vi "Supplementary Fig.13.vi"() -> ()   [LabVIEW 2018]
uses:
  <vilib>/Utility/miscctls.llb/LVBoundsTypeDef.ctl
panel:
  out "files":string[](array[string])=["3rd-no3_th0_20191112171700-ext.FIRE", "3rd-no3_th0_20191112171706-ext.FIRE", "3rd-no3_th0_20191112171712-ext.FIRE", "3rd-no3_th0_20191112171717-ext.FIRE", "3rd-no3_th0_20191112171723-ext.FIRE", "3rd-no3_th0_20191112171728-ext.FIRE", "3rd-no3_th0_20191112171733-ext.FIRE", "3rd-no3_th0_20191112171739-ext.FIRE", "3rd-no3_th0_20191112171744-ext.FIRE", "3rd-no3_th0_20191112171750-ext.FIRE", "3rd-no3_th0_20191112171756-ext.FIRE", "3rd-no3_th0_20191112171801-ext.FIRE", "3rd-no3_th0_20191112171807-ext.FIRE", "3rd-no3_th0_20191112171813-ext.FIRE", "3rd-no3_th0_20191112171819-ext.FIRE", "3rd-no3_th0_20191112171824-ext.FIRE", "3rd-no3_th0_20191112171829-ext.FIRE", "3rd-no3_th0_20191112171835-ext.FIRE", "3rd-no3_th0_20191112171840-ext.FIRE", "3rd-no3_th0_20191112171846-ext.FIRE", "3rd-no3_th0_20191112171851-ext.FIRE", "3rd-no3_th0_20191112171857-ext.FIRE"]
  out "current frame":i32=124
  out "N of files":i32=10
  out "N of frames":i32=1847
  out "current file index":i32
  in  "show imgs":bool=TRUE
  out "appended path":path
  in  "file type":string=".FIRE"
  in  "review all files":bool=TRUE
  in  "filepath":path
  out "radius [pixels]":dbl=1.3550767866040332
  out "Waveform Graph 2":dbl[][](graph)=[[262.50887727922697, 262.50887727922697, 262.50887727922697, 262.50887727922697, 262.50887727922697, 262.50887727922725, 262.50887727927375, 262.5088772849018, 262.5088777524451, 262.50890442157873, 262.50994809486673, 262.53793510133295, 263.05124338288414, 269.47198545530205, 323.99751463890766, 635.9891946850557, 1822.8576851199607, 4746.417892476711, 9125.351007955644, 12312.045868820023, 11530.560524463535, 7510.345954889637, 3469.141006273889, 1238.3317215458437, 466.76446485409394, 291.9163724708254, 265.4210910245801, 262.7072443516524, 262.5181711588755, 262.5091767852969, 262.50888391811486, 262.5088773804469, 262.50887728028846, 262.50887727923464, 262.508877279227, 262.50887727922697, 262.50887727922697, 262.50887727922697, 262.50887727922697, 262.50887727922697], [0.0, 0.0, 156.0, 214.0, 176.0, 193.0, 196.0, 216.0, 242.0, 278.0, 248.0, 395.0, 378.0, 505.0, 677.0, 1075.0, 1919.0, 4366.0, 9119.0, 12700.0, 11223.0, 7493.0, 3460.0, 1583.0, 638.0, 515.0, 344.0, 248.0, 266.0, 272.0, 252.0, 198.0, 173.0, 199.0, 174.0, 146.0, 153.0, 157.0, 149.0, 139.0]]
  out "Waveform Graph":dbl[][](graph)=[[174.75525223178883, 174.75525223178883, 174.75525223178883, 174.75525223178883, 174.75525223178883, 174.75525223178883, 174.75525223178883, 174.75525223178883, 174.75525223178883, 174.75525223178883, 174.75525223178883, 174.75525223178883, 174.75525223178883, 174.75525223178883, 174.75525223178883, 174.75525223178883, 174.75525223178883, 174.75525223178883, 174.75525223178883, 174.75525223178883, 174.75525223178883, 174.75525223178883, 174.75525223178883, 174.75525223178883, 174.75525223178883, 174.75525223178883, 174.75525223178883, 174.75525223178883, 174.75525223178883, 174.75525223178883, 174.7552522317898, 174.75525223221243, 174.75525233976546, 174.7552681981292, 174.7566217479153, 174.82339426848142, 176.72200269754504, 207.68357465442986, 494.55354551253936, 1976.3987968941556, 6062.483958450554, 11336.00697874787, 12448.136024265812, 8003.672547569417, 3071.60116130935, 796.5331441294701, 252.17136307296266, 180.3465628011094, 174.98950356645182, 174.76094517333206, 174.75533248779928, 174.75525288809214, 174.75525223490212, 174.75525223179739, 174.75525223178883, 174.75525223178883, 174.75525223178883, 174.75525223178883, 174.75525223178883, 174.75525223178883, 174.75525223178883, 174.75525223178883, 174.75525223178883, 174.75525223178883, 174.75525223178883, 174.75525223178883, 174.75525223178883, 174.75525223178883, 174.75525223178883, 174.75525223178883, 174.75525223178883, 174.75525223178883, 174.75525223178883, 174.75525223178883, 174.75525223178883, 174.75525223178883, 174.75525223178883, 174.75525223178883, 174.75525223178883, 174.75525223178883, 174.75525223178883, 174.75525223178883, 174.75525223178883, 174.75525223178883, 174.75525223178883, 174.75525223178883, 174.75525223178883, 174.75525223178883], [106.0, 109.0, 111.0, 109.0, 116.0, 100.0, 109.0, 105.0, 118.0, 105.0, 119.0, 114.0, 117.0, 123.0, 152.0, 136.0, 111.0, 148.0, 141.0, 156.0, 147.0, 159.0, 168.0, 147.0, 158.0, 143.0, 174.0, 193.0, 154.0, 196.0, 167.0, 197.0, 224.0, 252.0, 343.0, 365.0, 405.0, 565.0, 988.0, 2204.0, 5923.0, 11180.0, 12700.0, 7944.0, 2764.0, 1135.0, 731.0, 486.0, 419.0, 334.0, 249.0, 223.0, 190.0, 167.0, 167.0, 154.0, 147.0, 157.0, 143.0, 145.0, 140.0, 152.0, 157.0, 144.0, 150.0, 141.0, 126.0, 134.0, 145.0, 133.0, 105.0, 122.0, 120.0, 127.0, 131.0, 117.0, 100.0, 100.0, 96.0, 110.0, 110.0, 100.0, 107.0, 98.0, 102.0, 109.0, 0.0, 0.0]]
  in  "Threshold Limits 2":cluster{"Lower value":sgl, "Upper value":sgl}={"Lower value"=20.0, "Upper value"=60005.0} {"Upper value" format="%.2f"; "Lower value" format="%.2f"}
  in  "Threshold Limits":cluster{"Lower value":sgl, "Upper value":sgl}={"Lower value"=50.0, "Upper value"=60000.0} {"Upper value" format="%.2f"; "Lower value" format="%.2f"}
  in  "input 2":T1={"Niblack Dev Fac"=0.6000000000000001, "Window"={"Width"=50, "Height"=50}, "Sauvola Dev Rng"=2.0, "adaptive"=FALSE, "Method (Niblack)"=1} {"Method (Niblack)" items=["Niblack", "Background Correction", "Sauvola"]}
  in  "in1":T1={"Niblack Dev Fac"=0.5, "Window"={"Width"=20, "Height"=20}, "Sauvola Dev Rng"=6000.0, "adaptive"=FALSE, "Method (Niblack)"=0} {"Method (Niblack)" items=["Niblack", "Background Correction", "Sauvola"]}
  in  "post proc 2":T2={"trunc for ch2 masking"=[2, 2, 5, 2], "Erosion(pre)"=2, "Op"=enum."PClose", "post proc"=TRUE, "move x/y"=[0, 0], "conv"=FALSE, "Conn"=TRUE, "iterations"=5, "Erosion(post)"=2}
  in  "post proc1":T3={"trunc for ch2 masking"=[0, 0, 0, 0], "Erosion(pre)"=2, "Op"=enum."PClose", "post proc"=FALSE, "move x/y"=[0, 0], "conv"=TRUE, "Conn"=TRUE, "iteration"=5, "Erosion(post)"=2}
  in  "seg meth 2":T4={"norm for thresh"=TRUE, "use thresh formula"=FALSE, "thresh"=0.27000000000000013, "man thresh"=FALSE, "Meth"=0, "upper lim"=65000} {"Meth" items=["clustering", "entropy", "metric", "moments", "inter-class variance"]; "thresh" format="%_3g"}
  in  "seg meth":T4={"norm for thresh"=TRUE, "use thresh formula"=FALSE, "thresh"=0.2999999999995926, "man thresh"=TRUE, "Meth"=0, "upper lim"=64100} {"Meth" items=["clustering", "entropy", "metric", "moments", "inter-class variance"]; "thresh" format="%_3g"}
  in  "lpf 2":cluster{"cut":dbl, "lpf":bool, "odr":i32}={"cut"=0.2900001, "lpf"=FALSE, "odr"=2} {"cut" min=1e-07 max=0.4999 step=0.01 format="%_2g"}
  in  "lpf 1":cluster{"cut":dbl, "lpf":bool, "odr":i32}={"cut"=0.15000010000000014, "lpf"=FALSE, "odr"=2} {"cut" min=1e-07 max=0.4999 step=0.01 format="%_2g"}
  in  "save data":bool=TRUE
  in  "scale fac1":dbl=1.0000000000000009 min=0.01 max=10.0 step=0.01 format="%_3g"
  in  "scale fac2":dbl=0.9999999999999983 min=0.01 max=10.0 step=0.01 format="%_3g"
  in  "autoscale":bool=TRUE
  out "ch1":picture
  out "ch2":picture
  in  "color":T5(array[cluster])=[{"color array"=[0, 16711680, 16776960, 16448250, 65280, 16776960, 16711680, 16448250, 16448250], "num of colors"=2, "max"=4900.0, "min"=-1.0}, {"color array"=[0, 6618880, 16776960, 16448250, 65280, 16776960, 16711680, 16448250, 16448250], "num of colors"=2, "max"=9000.0, "min"=0.0}, {"color array"=[0, 255, 16448250, 16448250, 16776960, 16711680, 16448250, 16448250], "num of colors"=2, "max"=1.0, "min"=0.0}] {"min" step=0.01 format="%_2f"; "max" step=0.1 format="%_3f"}
  out "max2":dbl=12700.0
  out "max1":dbl=21856.0
  in  "Draw Area Size":T6
  in  "zoom":dbl=1.9999999999999973 format="%_2g"
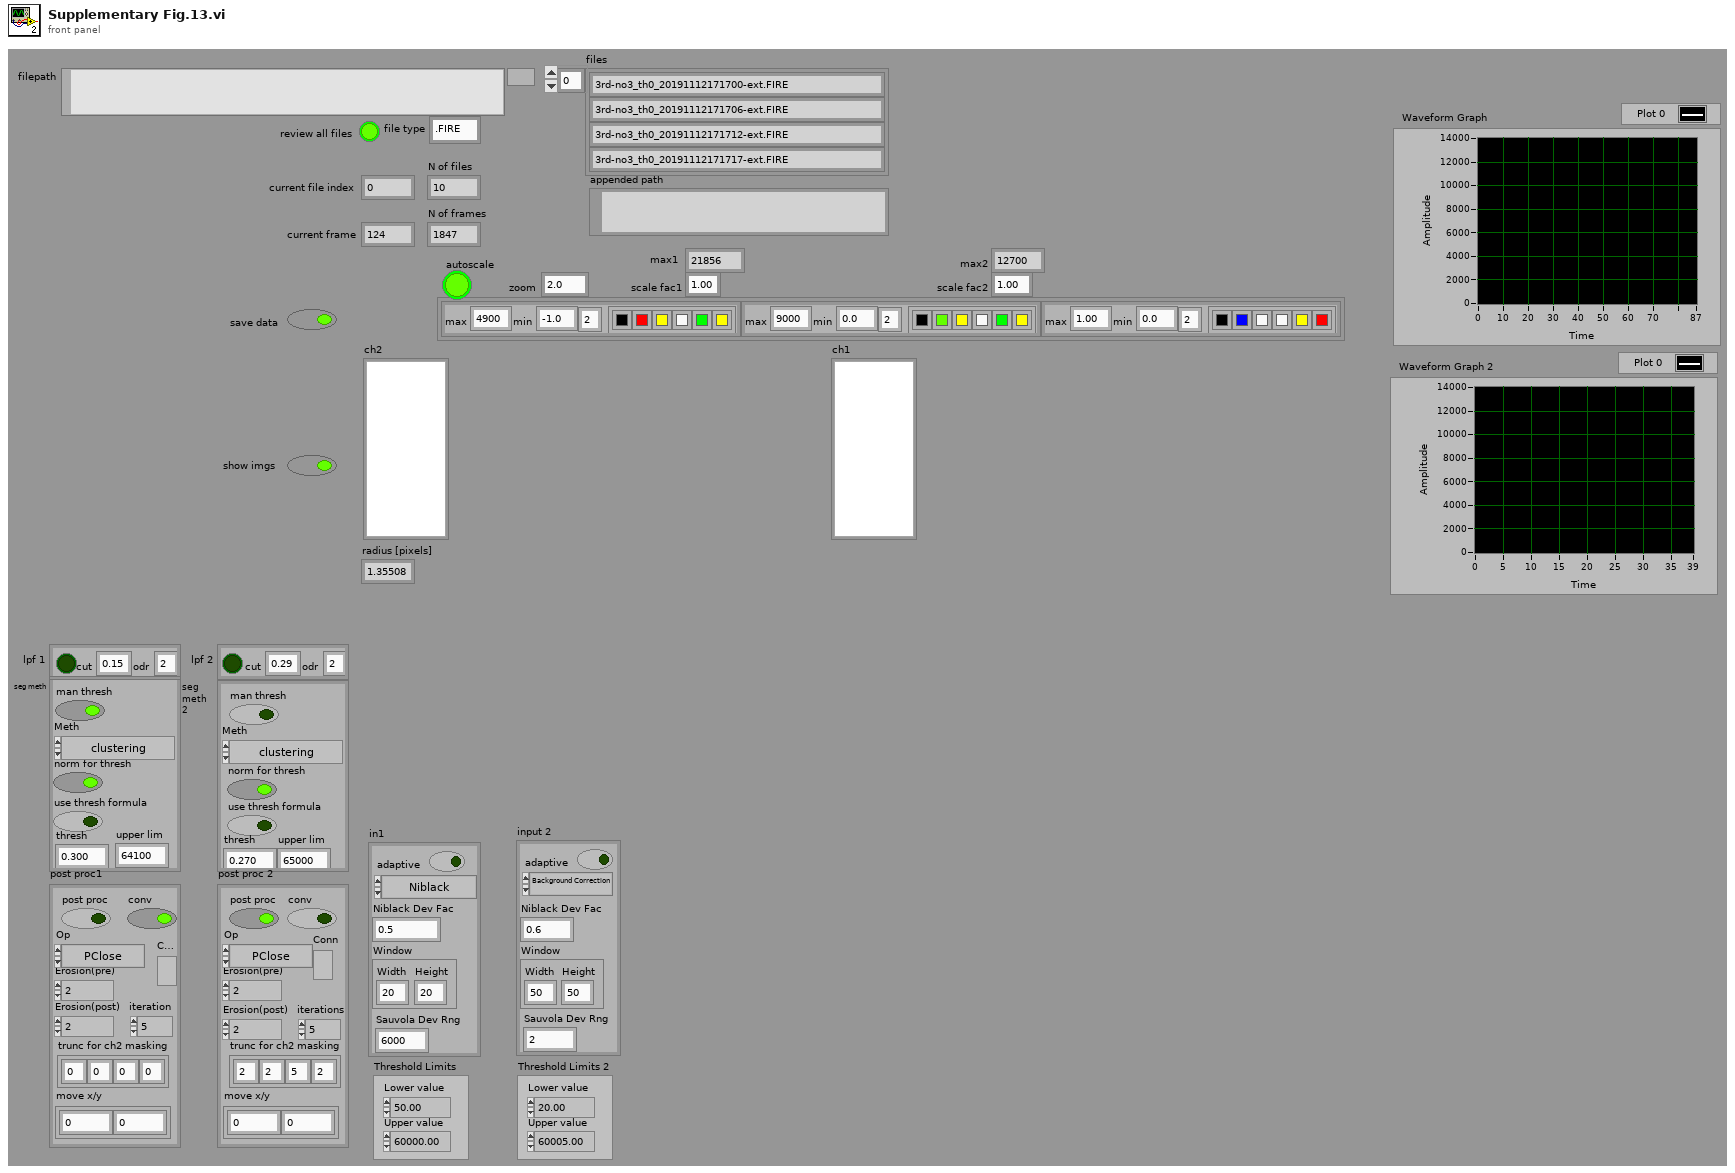
[diagram p1: front panel]
types:
  T1 = cluster{"Niblack Dev Fac":dbl, "Window":cluster{"Width":i32, "Height":i32}, "Sauvola Dev Rng":dbl, "adaptive":bool, "Method (Niblack)":u32}
  T2 = cluster{"trunc for ch2 masking":i32[], "Erosion(pre)":i32, "Op":enum32{"AutoM", "Close", "Dilate", "Erode", "Gradient", "Gradient out", "Gradient in", "Hit miss", "Open", "PClose", "POpen", "Thick", "Thin"}, "post proc":bool, "move x/y":i32[], "conv":bool, "Conn":bool, "iterations":i32, "Erosion(post)":i32}
  T3 = cluster{"trunc for ch2 masking":i32[], "Erosion(pre)":i32, "Op":enum32{"AutoM", "Close", "Dilate", "Erode", "Gradient", "Gradient out", "Gradient in", "Hit miss", "Open", "PClose", "POpen", "Thick", "Thin"}, "post proc":bool, "move x/y":i32[], "conv":bool, "Conn":bool, "iteration":i32, "Erosion(post)":i32}
  T4 = cluster{"norm for thresh":bool, "use thresh formula":bool, "thresh":dbl, "man thresh":bool, "Meth":i32, "upper lim":i32}
  T5 = cluster{"color array":u32[], "num of colors":i32, "max":dbl, "min":dbl}[]
  T6 = typedef "LVBoundsTypeDef.ctl" = cluster{"Width":u32, "Height":u32}
  T7 = enum16{"open", "replace", "create", "open or create", "replace or create", "replace or create with confirmation"}
  T8 = cluster{"color array":u32[], "num of colors":i32, "max":dbl, "min":dbl}
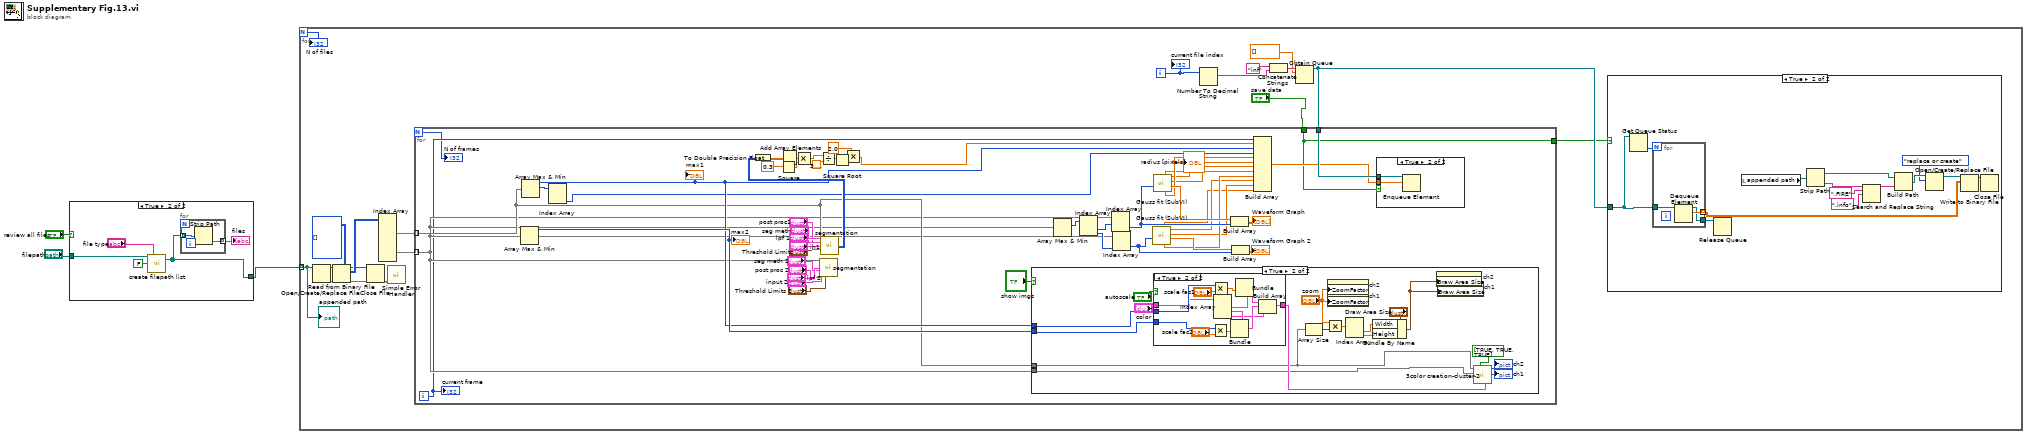
[diagram p0: block diagram]
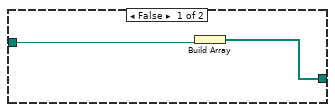
[diagram p2: hidden frame]
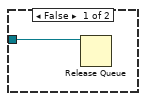
[diagram p6: hidden frame]
diagram:
  n1 = case shown="True" "review all files" {
    tunnel: "filepath" -> [w5 w8]
    tunnel: [w4 w6] -> w1
    frame False {
      n2 = Build Array(w5) -> (w4:path[])
    }
    frame True {
      n3 = call "create filepath list.vi"("regular expression"="file type", "search subholder"=FALSE, "path"=w8) -> ("Array"=w6:path[])  [unwired: 1 out]
      n4 = for {
        tunnel: w6 -> [w12] mode=indexing
        tunnel: [w11] -> w7 mode=indexing
        n5 = Strip Path(path=w12) -> (name=w11:string)  [unwired: 1 out]
      }
      "files" <- w7
    }
  }
  n6 = for {
    N -> [w14]
    tunnel: w1 -> [w16] mode=indexing
    i -> [w15]
    n7 = Open/Create/Replace File(file path (use dialog)=w16) -> (refnum out=w24:refnum<file>, error out=w23:errorcluster)  [unwired: 5 in, 1 out]
    n8 = Read from Binary File(5:i32[][][][] [], 8:w23, 11:w24) -> (0:w21:errorcluster, 2:w25:i32[][][][], 3:w20:refnum<file>)  [unwired: 3 in, 1 out]
    n9 = Close File(refnum=w20, error in=w21) -> (error out=w22:errorcluster)  [unwired: 1 out]
    n10 = Index Array(array=w25) -> (element #1=w18:i32[][][], element #2=w17:i32[][][])  [unwired: 8 in]
    n11 = call <vilib>:"Simple Error Handler.vi"("error in (no error)"=w22) -> ()  [unwired: 4 in, 5 out]
    n12 = Number To Decimal String(number=w15) -> (decimal integer string=w28:string)  [unwired: 1 in]
    n13 = Concatenate Strings("inf" ("name (unnamed)"), w28) -> (w29:string)
    n14 = Obtain Queue(name (unnamed)=w29, element data type=dbl[] [] ("Array")) -> (queue out=w30:refnum<queue>)  [unwired: 3 in, 2 out]
    n15 = for {
      N -> [w33]
      tunnel: w30 -> [w70]
      tunnel: "save data" -> [w32]
      tunnel: w18 -> [w36] mode=indexing
      tunnel: w17 -> [w35] mode=indexing
      tunnel: [w32] -> w13
      i -> [w34]
      n16 = Array Max & Min(array=w35) -> (max value=w73:i32)  [unwired: 3 out]
      "max2" <- w73
      n17 = Array Max & Min(array=w36) -> (max value=w58:i32, max index (indices)=w57:i32[])  [unwired: 2 out]
      "max1" <- w58
      n18 = Index Array(array=w57) -> (element #2=w56:i32)  [unwired: 2 in, 1 out]
      n19 = Square(x=0.3) -> (x^2=w66:dbl)
      n20 = call "segmentation.vi"("unmixed ch2"=w35, "segmentation method"="seg meth 2", "image lpf"="lpf 2", "post processing"="post proc 2", "input cluster"="input 2", "Threshold Limits"="Threshold Limits 2") -> ()  [unwired: 7 in, 3 out]
      n21 = call "segmentation.vi"("unmixed ch2"=w36, "segmentation method"="seg meth", "image lpf"="lpf 1", "post processing"="post proc1", "input cluster"="in1", "Threshold Limits"="Threshold Limits") -> ("Array"=w69:u8[][])  [unwired: 7 in, 2 out]
      n22 = To Double Precision Float(number=w69) -> (double precision float=w60:dbl[][])
      n23 = Add Array Elements(numeric array=w60) -> (sum=w68:dbl)
      n24 = Multiply(x=w68, y=w66) -> (x*y=w65:dbl)
      n25 = Divide(x=w65, y=3.141592653589793) -> (x/y=w63:dbl)
      n26 = Square Root(x=w63) -> (sqrt(x)=w62:dbl)
      n27 = Multiply(x=2.0, y=w62) -> (x*y=w59:dbl)
      n28 = case shown="True" "show imgs" {
        tunnel: w36 -> [_ w85]
        tunnel: w35 -> [_ w84]
        tunnel: w73 -> [_ w92]
        tunnel: w58 -> [_ w91]
        frame False {
        }
        frame True {
          n29 = case shown="True" "autoscale" {
            tunnel: w91 -> [_ w112]
            tunnel: w92 -> [_ w111]
            tunnel: "color" -> [w101 w108]
            tunnel: [w101 w107] -> w90
            frame False {
            }
            frame True {
              n30 = Multiply(x=w111, y="scale fac2") -> (x*y=w105:dbl)
              n31 = Multiply(x=w112, y="scale fac1") -> (x*y=w106:dbl)
              n32 = Index Array(array=w108) -> (element #1=w114:T8, element #2=w113:T8, element #3=w102:T8)  [unwired: 3 in]
              n33 = Bundle(cluster=w113, "max"=w105) -> (w109:T8)  [unwired: 3 in]
              n34 = Bundle(cluster=w114, "max"=w106) -> (w110:T8)  [unwired: 3 in]
              n35 = Build Array(w110, w109, w102) -> (w107:T5)
            }
          }
          n36 = Array Size(array=w85) -> (size(s)=w93:i32[])
          n37 = Multiply(x="zoom", y=w93) -> (x*y=w94:dbl[])
          n38 = property on="ch2" class="Pict"("ZoomFactor"="zoom") -> ()  [unwired: 2 in, 2 out]
          n39 = property on="ch1" class="Pict"("ZoomFactor"="zoom") -> ()  [unwired: 2 in, 2 out]
          n40 = Index Array(array=w94) -> (element #1=w86:dbl, element #2=w87:dbl)  [unwired: 2 in]
          n41 = Bundle By Name(cluster="Draw Area Size", "Width"=w86, "Height"=w87) -> (w97:T6)
          n42 = property on="ch2" class="Pict"("Draw Area Size"=w97) -> ()  [unwired: 2 in, 2 out]
          n43 = property on="ch1" class="Pict"("Draw Area Size"=w97) -> ()  [unwired: 2 in, 2 out]
          n44 = call "3color creation-cluster-2.vi"("color"=w90, "Array 4"=bool[] [TRUE, TRUE, TRUE], "Array 2"=w84, "Array"=w85) -> ("ch2"=→"ch1":picture, "ch1"=→"ch2":picture)  [unwired: 2 in, 2 out]
        }
      }
      n45 = Array Max & Min(array=w35) -> (max index (indices)=w53:i32[])  [unwired: 3 out]
      n46 = Index Array(array=w53) -> (element #1=w52:i32, element #2=w51:i32)  [unwired: 2 in]
      n47 = Index Array(array=w35, index (row)=w52) -> (element=w49:i32[])  [unwired: 1 in]
      n48 = Index Array(array=w35, index (col)=w51) -> (element=w47:i32[])  [unwired: 1 in]
      n49 = call "Gauss fit (SubVI).vi"("Array"=w47) -> ("Best Gaussian Fit"=w46:dbl[], "amplitude"=w38:dbl, "center"=w39:dbl, "standard deviation"=w40:dbl, "residue"=w37:dbl)  [unwired: 5 in, 1 out]
      n50 = call "Gauss fit (SubVI).vi"("Array"=w49) -> ("Best Gaussian Fit"=w48:dbl[], "amplitude"=w43:dbl, "center"=w42:dbl, "standard deviation"=w44:dbl, "residue"=w41:dbl)  [unwired: 5 in, 1 out]
      "radius [pixels]" <- w44
      n51 = Build Array(w48, w49) -> (→"Waveform Graph":dbl[][])
      n52 = Build Array(w46, w47) -> (→"Waveform Graph 2":dbl[][])
      n53 = Build Array(w34, w59, w58, w56, w44, w43, w42, w41, w40, w39, w38, w37) -> (w54:dbl[])
      n54 = case shown="True" w32 {
        tunnel: w70 -> [_ w83]
        tunnel: w54 -> [_ w82]
        frame False {
        }
        frame True {
          n55 = Enqueue Element(queue=w83, element=w82) -> ()  [unwired: 2 in, 3 out]
        }
      }
      "N of frames" <- w33
      "current frame" <- w34
    }
    n56 = case shown="True" w13 {
      tunnel: w30 -> [w115 w122]
      frame False {
        n57 = Release Queue(queue=w115) -> ()  [unwired: 2 in, 3 out]
      }
      frame True {
        n58 = Get Queue Status(queue=w122) -> (# elements in queue=w126:i32)  [unwired: 2 in, 7 out]
        n59 = for {
          N: w126 -> [_]
          tunnel: w122 -> [w132]
          tunnel: [w131] -> w121 mode=indexing
          tunnel: [w130] -> w125
          n60 = Dequeue Element(queue=w132) -> (queue out=w130:refnum<queue>, element=w131:dbl[])  [unwired: 2 in, 2 out]
        }
        n61 = Release Queue(queue=w125) -> ()  [unwired: 2 in, 3 out]
        n62 = local read "appended path"() -> (w118:path)
        n63 = Strip Path(path=w118) -> (stripped path=w116:path, name=w119:string)
        n64 = Search and Replace String(input string=w119, search string=".FIRE" ("substring (\"\")"), replace string=".info" ("replace string (\"\")")) -> (result string=w117:string)  [unwired: 5 in, 3 out]
        n65 = Build Path(base path=w116, name or relative path=w117) -> (appended path=w127:path)
        n66 = Open/Create/Replace File(file path (use dialog)=w127, operation (0:open)=T7."replace or create") -> (refnum out=w128:refnum<file>)  [unwired: 4 in, 2 out]
        n67 = Write to Binary File(file (use dialog)=w128, data=w121) -> (refnum out=w129:refnum<file>)  [unwired: 4 in, 2 out]
        n68 = Close File(refnum=w129) -> ()  [unwired: 1 in, 2 out]
      }
    }
    "appended path" <- w16
    "current file index" <- w15
    "N of files" <- w14
  }
